vi "Highlight Item.vi"(8 "error in":errorcluster, 10 "Tag":string, 11 "TreeControl in":refnum<vi>) -> (0 "error out":errorcluster, 3 "TreeControl out":refnum<vi>)   [LabVIEW 2019, in "Panther Dashboard.lvlib"]
uses:
  Panther Dashboard.lvlib
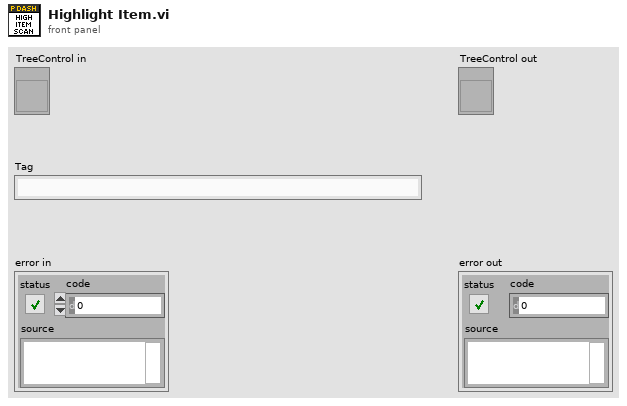
[diagram p1: front panel]
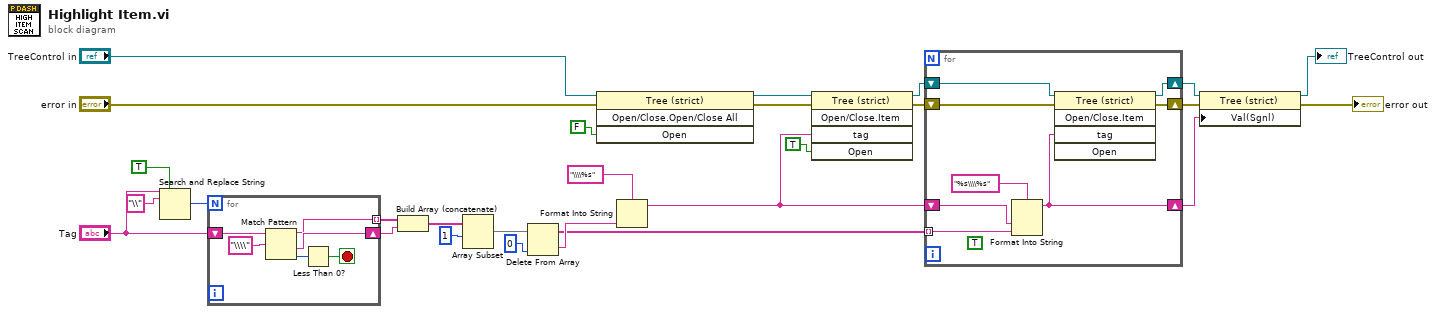
[diagram p0: block diagram]
diagram:
  n1 = Search and Replace String(replace all?=TRUE ("replace all? (F)"), input string="Tag", search string="\\") -> (number of replacements=w20:i32)  [unwired: 5 in, 3 out]
  n2 = for {
    N: w20 -> [_]
    tunnel: [w28] -> w19 mode=indexing
    shift-right: [w29] -> w18
    shift-left: "Tag" -> [w33]
    stop <- w30 stop-if-true
    n3 = Match Pattern(string=w33, regular expression="\\\\" ("search string")) -> (before substring=w28:string, after substring=w29:string, offset past match=w31:i32)  [unwired: 1 in, 1 out]
    n4 = Less Than 0?(x=w31) -> (x < 0?=w30:bool)
  }
  n5 = Build Array (concatenate)(w19, w18) -> (w17:string[])
  n6 = Array Subset(array=w17, index=1) -> (w14:string[])  [unwired: 1 in]
  n7 = Delete From Array(array=w14, index=0) -> (deleted portion=w13:string, array with subset deleted=w11:string[])  [unwired: 1 in]
  n8 = invoke class="Tree (strict)" method="Open/Close.Open/Close All"(reference="TreeControl in", error in="error in", "Open"=FALSE ("Open?")) -> (reference out=w7:refnum<vi>, error out=w25:errorcluster)  [unwired: 1 in, 2 out]
  n9 = Format Into String(format string="\\\\%s", w13) -> (resulting string=w5:string)  [unwired: 2 in, 1 out]
  n10 = invoke class="Tree (strict)" method="Open/Close.Item"(reference=w7, error in=w25, "tag"=w5, "Open"=TRUE ("Open?")) -> (reference out=w6:refnum<vi>, error out=w24:errorcluster)  [unwired: 1 in, 3 out]
  n11 = for {
    tunnel: w11 -> [w36] mode=indexing
    shift-right: [w34] -> w1
    shift-left: w5 -> [w37]
    shift-right: [w40] -> w26
    shift-left: w24 -> [w41]
    shift-right: [w38] -> w3
    shift-left: w6 -> [w39]
    (unwired) TRUE ("Open?")
    n12 = Format Into String(format string="%s\\\\%s", w37, w36) -> (resulting string=w34:string)  [unwired: 2 in, 1 out]
    n13 = invoke class="Tree (strict)" method="Open/Close.Item"(reference=w39, error in=w41, "tag"=w34) -> (reference out=w38:refnum<vi>, error out=w40:errorcluster)  [unwired: 2 in, 3 out]
  }
  n14 = property class="Tree (strict)"(reference=w3, error in=w26, "Val(Sgnl)"=w1) -> (reference out=→"TreeControl out":refnum<vi>, error out=→"error out":errorcluster)
